vi "asAcq_dataWaitGet.vi"(0 "reference":refnum<class "OSA300.lvclass">, 2 "dataType":T1=enum."interferogram", 5 "error in (no error)":errorcluster, 7 "timeout (20000 ms)":i32=60000, 9 "error if timeout":bool=TRUE, 11 "ignore interfrgrm wLmt (OSA300)":bool=TRUE) -> (13 "timeOut":bool, 14 "duplicate reference":refnum<class "OSA300.lvclass">, 16 "dataType out":T1=enum."interferogram", 19 "error out":errorcluster)   [LabVIEW 2010, in "OSA300.lvclass"]
doc: "Waits for new data to be available and store retrieved data in a labview buffer, (see buffer_get.vi for data access)."
uses:
  OSA300.lvclass
  typeDef/acq_dataType.ctl
  OSA.lvclass
  OSA20X_misc.lvlib
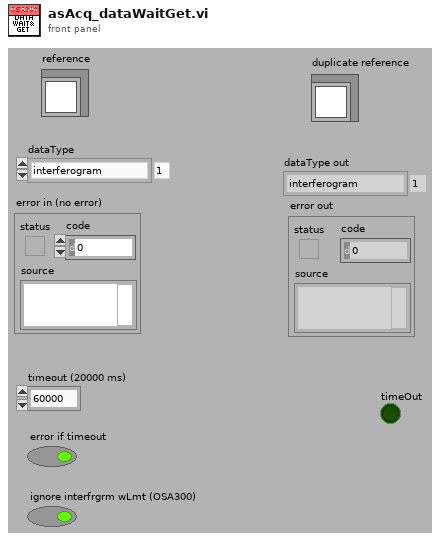
[diagram p1: front panel]
types:
  T1 = typedef "OSA.lvclass/acq_dataType.ctl" = enum16{"none", "interferogram", "spectrum"}
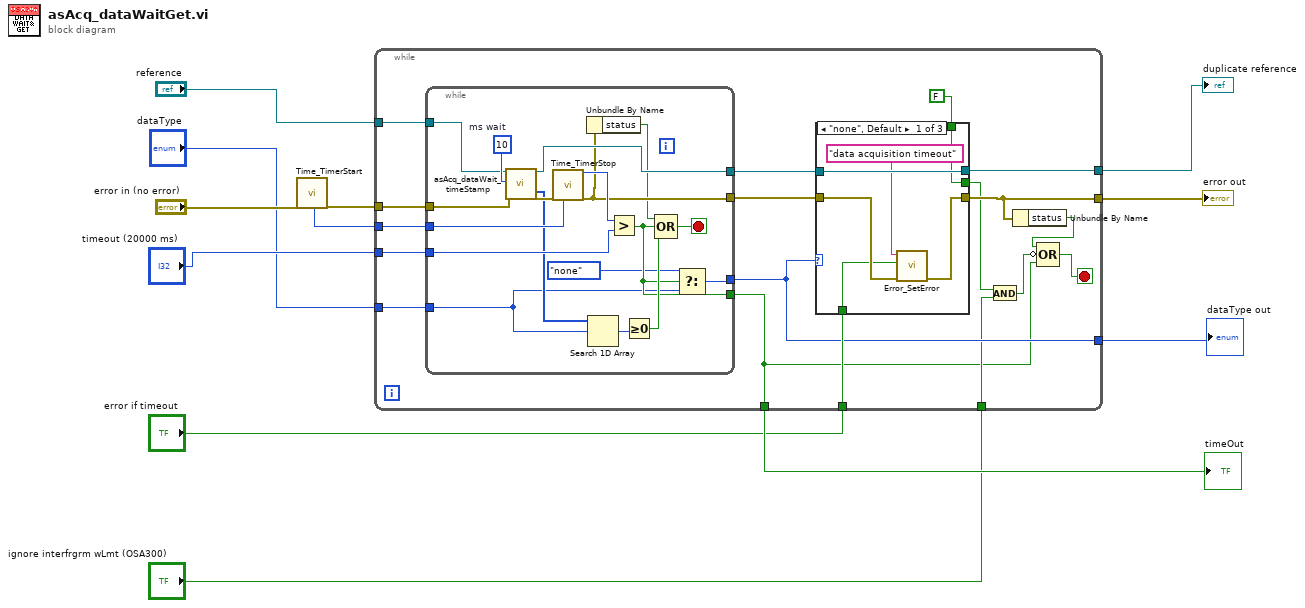
[diagram p0: block diagram]
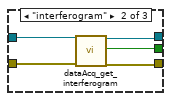
[diagram p2: hidden frame]
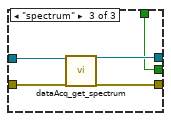
[diagram p3: hidden frame]
diagram:
  n1 = call "Time_TimerStart.vi"("error in (no error)"="error in (no error)") -> ("Start Value (ms timer)"=w11:u32, "error out"=w12:errorcluster)  [unwired: 17 in]
  n2 = while {
    tunnel: w12 -> [w28]
    tunnel: w11 -> [w27]
    tunnel: "reference" -> [w26]
    tunnel: [w25] -> w9
    tunnel: "timeout (20000 ms)" -> [w24]
    tunnel: "dataType" -> [w23]
    tunnel: [w14] -> w5
    tunnel: "error if timeout" -> [w22]
    tunnel: [w21] -> w3
    tunnel: [w20] -> w2
    tunnel: "ignore interfrgrm wLmt (OSA300)" -> [w19]
    stop <- w15 stop-if-true
    n3 = while {
      tunnel: [w48] -> w30
      tunnel: [w61] -> w29
      tunnel: w28 -> [w64]
      tunnel: w27 -> [w60]
      tunnel: w24 -> [w58]
      tunnel: w23 -> [w49]
      tunnel: w26 -> [w55]
      tunnel: [w52] -> w21
      tunnel: [w51] -> w14
      stop <- w54 stop-if-true
      w63 = 10  # ms wait
      n4 = call "asAcq_dataWait_timeStamp.vi"("reference"=w55, "ms wait"=w63, "error in (no error)"=w64) -> ("duplicate reference"=w61:refnum<class "OSA300.lvclass">, "dataType"=w57:T1[], "error out"=w62:errorcluster)  [unwired: 14 in]
      n5 = call "Time_TimerStop.vi"("error in (no error)"=w62, "Start Value (millisecond timer)"=w60) -> ("Time (millisecond timer)"=w59:i32, "error out"=w48:errorcluster)  [unwired: 16 in]
      n6 = Unbundle By Name(w48) -> ("status"=w47:bool)
      n7 = Search 1D Array(1D array=w57, element=w49) -> (index of element=w56:i32)  [unwired: 1 in]
      n8 = Greater?(x=w59, y=w58) -> (0:w51:bool)
      n9 = Greater Or Equal To 0?(x=w56) -> (x >= 0?=w53:bool)
      n10 = Compound Arithmetic op=OR(w47, w51, w53) -> (w54:bool)
      n11 = Select(t=acq_dataType."none" ("dataType"), s=w51, f=w49) -> (s? t:f=w52:T1)
    }
    n12 = case shown="\"none\", Default" w21 {
      tunnel: w29 -> [w36 w38 w46]
      tunnel: w30 -> [w34 w41 w45]
      tunnel: [w33 w40 w44] -> w20
      tunnel: [w36 w39 w43] -> w25
      tunnel: w22 -> [w32 _ _]
      tunnel: [w31 w37 w42] -> w18
      tunnel: FALSE ("saturated") -> [w31 _ w42]
      frame "none", Default {
        n13 = call "Error_SetError.vi"("error in"=w34, "status (true)"=w32, "source(\"\")"="data acquisition timeout" ("source(\"\")")) -> ("error out"=w33:errorcluster)  [unwired: 4 in]
      }
      frame "interferogram" {
        n14 = call-dynamic "dataAcq_get_interferogram.vi"("reference"=w38, "error in (no error)"=w41) -> ("duplicate reference"=w39:refnum<class "OSA300.lvclass">, "saturated"=w37:bool, "error out"=w40:errorcluster)  [unwired: 15 in]
      }
      frame "spectrum" {
        n15 = call-dynamic "dataAcq_get_spectrum.vi"("reference"=w46, "error in (no error)"=w45) -> ("duplicate reference"=w43:refnum<class "OSA300.lvclass">, "error out"=w44:errorcluster)  [unwired: 16 in]
      }
    }
    n16 = And(x=w18, y=w19) -> (x .and. y?=w16:bool)
    n17 = Unbundle By Name(w20) -> ("status"=w17:bool)
    n18 = Compound Arithmetic op=OR(w17, invert w16, w14) -> (w15:bool)
  }
  "error out" <- w2
  "duplicate reference" <- w9
  "timeOut" <- w5
  "dataType out" <- w3
